vi "qUSG SYS.vi"(0 "System no.":i32=1 min=1 max=4 step=1, 1 "Container Unit":string, 3 "Function Unit":string, 5 "error in":errorcluster) -> (14 "Unit Description List":T1[](array[typedef]), 19 "error out":errorcluster)   [LabVIEW 2026]
doc: "USG? SYS (System Overview)\n\nDescription \nOutputs the \"SYS\" section of the user guide.\nThe \"SYS\" section contains information on the structure of the controller, i.e. on the existing \ncontainer units and function units (p. 91). Depending on the argument(s) used, the display is \nlimited to certain units.\n\nFormat\nUSG? SYS[ <Container Unit>[ <Function Unit>]]\n\nArguments\n<Container Unit>\nContainer unit\nPossible values: Alias of the container unit (p. 94) \n<Function Unit>\nFunction unitIf <Function Unit> is not specified, information about all function units contained \nin the container unit are output.\nIf only information about a certain container unit are to be displayed, \"-\" must be entered for \n<Function Unit>.\nPossible values:\nAlias of the function unit (p. 94) \n\"-\" \n\nResponse\nThe output always has the following format:\nThe Unit Overview block consists of at least the following fields:\n- Container Unit Alias (p. 94) for the container unit\n- Function Unit Alias (p. 94) for the function unit. The value \"-\" means that the \ndescription refers to the container unit.\n- Description Description of the container unit or function unit.\n\nNotes\nUSG? without any arguments (p. 72) displays the contents of the user guide, i.e. the titles of the \navailable sections.\n\nUser command level\nUSR"
uses:
  UnitDescription.ctl
  <vilib>/Utility/error.llb/Trim Whitespace One-Sided.vi
panel:
  # "USG? SYS (System Overview)\n\nOutputs the \"SYS\" section of the user guide.\nThe \"SYS\" section contains information on the structure of the controller, i.e. on the existing container units and function units. Depending on the argument(s) used, the display is limited to certain units."
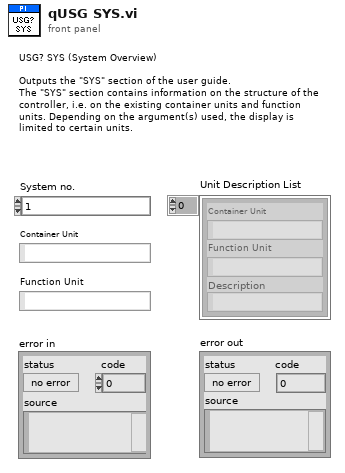
[diagram p1: front panel]
types:
  T1 = typedef "UnitDescription.ctl" = cluster{"Container Unit":string, "Function Unit":string, "Description":string}
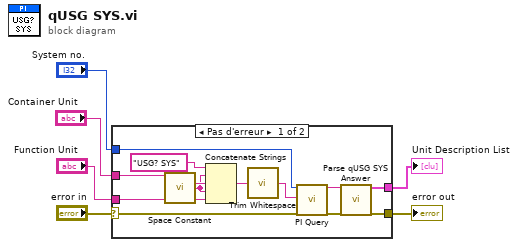
[diagram p0: block diagram]
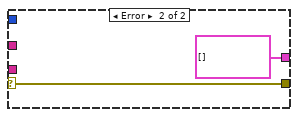
[diagram p2: hidden frame]
diagram:
  n1 = case shown="Pas d'erreur" "error in" {
    selector: "error in" -> [w18 w20]
    tunnel: "System no." -> [w17 _]
    tunnel: [w10 w20] -> w5
    tunnel: [w7 T1[] [] ("System Container Unit Description List")] -> w3
    tunnel: "Container Unit" -> [w13 _]
    tunnel: "Function Unit" -> [w14 _]
    frame No Error {
      n2 = call <vilib>:"Space Constant.vi"() -> ("String"=w12:string)
      n3 = Concatenate Strings("USG? SYS", w12, w13, w12, w14) -> (w15:string)
      n4 = call <vilib>:"Trim Whitespace.vi"("string"=w15) -> ("trimmed string"=w11:string)  [unwired: 1 in]
      n5 = call "PI Query.vi"("System no."=w17, "String to send"=w11, "error in"=w18) -> ("String read"=w8:string, "error out"=w9:errorcluster)  [unwired: 13 in, 2 out]
      n6 = call "Parse qUSG SYS Answer.vi"("Answer To Parse"=w8, "error in"=w9) -> ("Function Unit Info List"=w7:T1[], "error out"=w10:errorcluster)  [unwired: 16 in]
    }
    frame Error {
    }
  }
  "error out" <- w5
  "Unit Description List" <- w3
